vi "Ex2Task4_Main.vi"() -> ()   [LabVIEW 2014, in "Harper_3Ex2Task4.lvrbt"]
uses:
  C:/Users/ech6028/Documents/LabVIEW Data/NXTRobotics/Projects/Harper_3Ex2Task4/Harper_3Ex2Task4.lvrbt
  <vilib>/NXT/Block Support/NXT_InputPort.ctl
  <vilib>/NXT/Block Support/NXT_OutputPort.ctl
  <vilib>/NXT/Dual Mode Library/Sensors/EV3_Color_Ambient.vi
  <vilib>/NXT/NXTIO Xnodes/NXTIONodeSubVIs/NXTMoveMotors.vi
  <vilib>/NXT/Subs/LVHSConnector.ctl
  <vilib>/NXT/NXTIO Xnodes/AddressXNode/NXTIOAddress.xnode
  <vilib>/NXT/NXTIO Xnodes/NXTIOXNode/NXTIO.xnode
  <vilib>/NXT/LegoClasses/BrickReference/BrickReference.lvclass
panel:
  out "Sensor Value":sgl(graph)
  in  "stop":bool
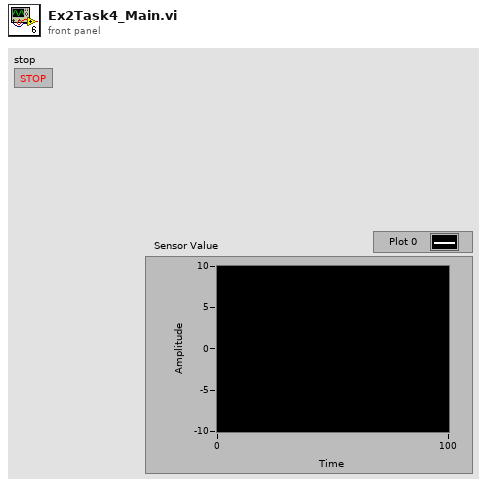
[diagram p1: front panel]
types:
  T1 = typedef "NXT_OutputPort.ctl" = u8
  T2 = typedef "NXT_InputPort.ctl" = u32
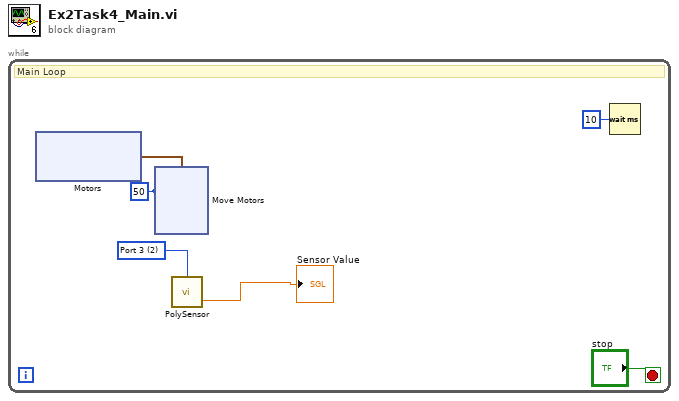
[diagram p0: block diagram]
diagram:
  n1 = while {
    stop <- "stop" stop-if-true
    w2 = T2 2 items=["Port 1", "Port 2", "Port 3", "Port 4"] ("Port (Port 1)")
    w3 = i8 50 ("Power/Speed 1")
    # "Main Loop"
    n2 = xnode "Motors"() -> ("Motor"=w4:cluster{"Port":T1, "Port":T1})
    n3 = xnode "Move Motors"("Power/Speed 2"=w3, "Power/Speed 1"=w3, "Motors"=w4) -> ()  [unwired: 1 in, 1 out]
    n4 = call-poly <vilib>:"PolySensor.vi"("Port (Port 1)"=w2) -> ("Scaled Value"=→"Sensor Value":sgl)  [unwired: 2 in, 1 out]
    n5 = Wait (ms)(milliseconds to wait=u32 10) -> ()  [unwired: 1 out]
  }
